vi "Get Measurement Library.vi"(7 "Error if not Found (T)":bool=TRUE, 8 "error in (no error)":errorcluster, 10 "Measurement Service Name":string, 11 "Project in":refnum<vi>) -> (0 "error out":errorcluster, 1 "Found":bool, 2 "Measurement Library Item":refnum<vi>)   [LabVIEW 2020, in "MeasurementService Editor.lvlib"]
uses:
  MeasurementService Editor.lvlib
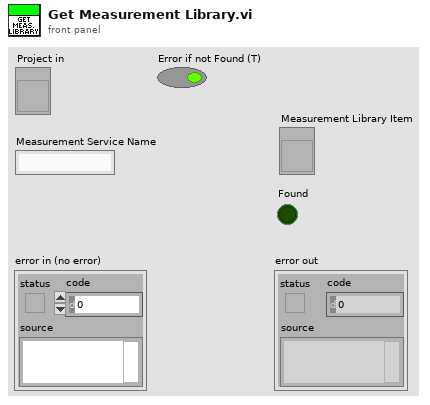
[diagram p1: front panel]
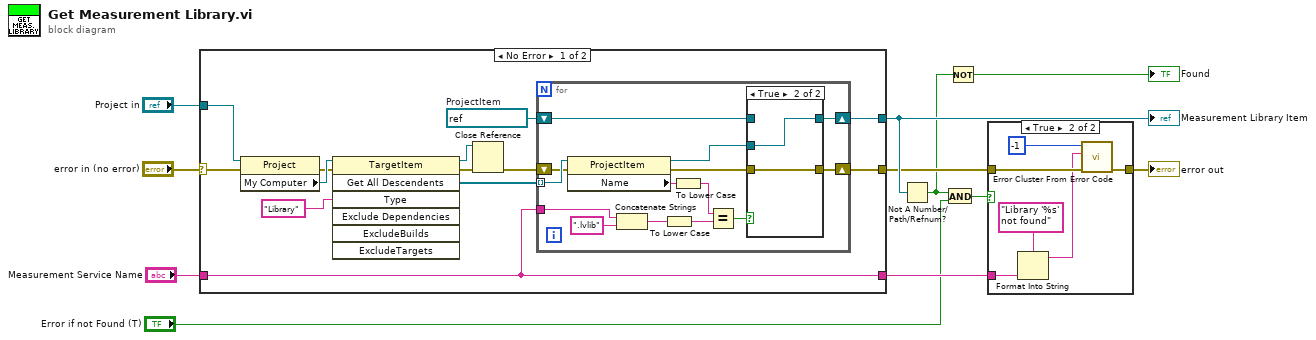
[diagram p0: block diagram]
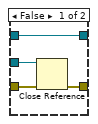
[diagram p3: hidden frame]
diagram:
  n1 = case shown="No Error" "error in (no error)" {
    selector: "error in (no error)" -> [w20 w46]
    tunnel: "Project in" -> [w24 _]
    tunnel: "Measurement Service Name" -> [w12 w45]
    tunnel: [w19 w46] -> w6
    tunnel: [w14 _] -> w8
    tunnel: [w12 w45] -> w5
    frame No Error {
      w15 = refnum<vi> refnum  # ProjectItem
      n2 = property class="Project"(reference=w24, error in=w20) -> (error out=w22:errorcluster, "My Computer"=w23:refnum<vi>)  [unwired: 1 out]
      n3 = invoke class="TargetItem" method="Get All Descendents"(reference=w23, error in=w22, "Type"="Library") -> (reference out=w17:refnum<vi>, error out=w18:errorcluster, "All Descendents"=w21:refnum<vi>[])  [unwired: 4 in, 4 out]
      n4 = Close Reference(reference=w17, error in (no error)=w18) -> (error out=w16:errorcluster)
      n5 = for {
        tunnel: w21 -> [w38] mode=indexing
        tunnel: w12 -> [w37]
        shift-right: [w31] -> w19
        shift-left: w16 -> [w35]
        shift-right: [w30] -> w14
        shift-left: w15 -> [w29]
        n6 = property class="ProjectItem"(reference=w38, error in=w35) -> (reference out=w33:refnum<vi>, error out=w34:errorcluster, "Name"=w26:string)
        n7 = Concatenate Strings(w37, ".lvlib" ("string")) -> (w28:string)
        n8 = To Lower Case(string=w28) -> (all lower case string=w27:string)
        n9 = To Lower Case(string=w26) -> (all lower case string=w25:string)
        n10 = Equal?(x=w25, y=w27) -> (x = y?=w32:bool)
        n11 = case shown="True" w32 {
          tunnel: w34 -> [w42 w44]
          tunnel: w33 -> [w39 w43]
          tunnel: [w41 w44] -> w31
          tunnel: [w40 w43] -> w30
          tunnel: w29 -> [w40 _]
          frame False {
            n12 = Close Reference(reference=w39, error in (no error)=w42) -> (error out=w41:errorcluster)
          }
          frame True {
          }
        }
      }
    }
    frame Error {
    }
  }
  "Measurement Library Item" <- w8
  n13 = Not A Number/Path/Refnum?(number/path/refnum=w8) -> (NaN/Path/Refnum?=w2:bool)
  n14 = And(x=w2, y="Error if not Found (T)") -> (x .and. y?=w4:bool)
  n15 = Not(x=w2) -> (.not. x?=→"Found":bool)
  n16 = case shown="True" w4 {
    tunnel: [w47 w53] -> w7
    tunnel: w6 -> [w47 w52]
    tunnel: w5 -> [_ w48]
    frame False {
    }
    frame True {
      n17 = Format Into String(format string="Library '%s' not found" ("initial string"), w48) -> (resulting string=w49:string)  [unwired: 2 in, 1 out]
      n18 = call <vilib>:"Error Cluster From Error Code.vi"("error in (no error)"=w52, "error message (\"\")"=w49, "error code (0)"=-1) -> ("error out"=w53:errorcluster)  [unwired: 6 in]
    }
  }
  "error out" <- w7
